vi "UpdateData_Wrapper.vi"(6 "50mA Spectra":cluster{"Wavelength":dbl[], "EL Spectrum":dbl[]}, 7 "20mA Spectra":cluster{"Wavelength":dbl[], "EL Spectrum":dbl[]}, 8 "error in (no error)":errorcluster, 10 "Data In":T1 {"50mA Data"."Reverse" format="%#_3g"; "50mA Data"."Current,mA" format="%_6g"; "50mA Data"."Knee Current" format="%#_3g"; "50mA Data"."WL" format="%_6g"; "50mA Data"."Voltage" format="%_6g"; "50mA Data"."Power" format="%_5g"; "20mA Data"."Reverse" format="%#_3g"; "20mA Data"."Current,mA" format="%_6g"; "20mA Data"."Knee Current" format="%#_3g"; "20mA Data"."WL" format="%_6g"; "20mA Data"."Voltage" format="%_6g"; "20mA Data"."Power" format="%_5g"}, 11 "EpiWrapper in":refnum<class "EpiWrapper.lvclass">) -> (0 "error out":errorcluster, 1 "PowerMin":dbl, 2 "KneeFail?":bool, 3 "EpiWrapper out":refnum<class "EpiWrapper.lvclass">)   [LabVIEW 2012, in "EpiWrapper.lvclass"]
uses:
  EpiWrapper.lvclass
  Controls/TestData.ctl
  Controls/Measurement.ctl
  EpiWrapper.lvclass/EpiWrapper.ctl
  LotData.lvclass
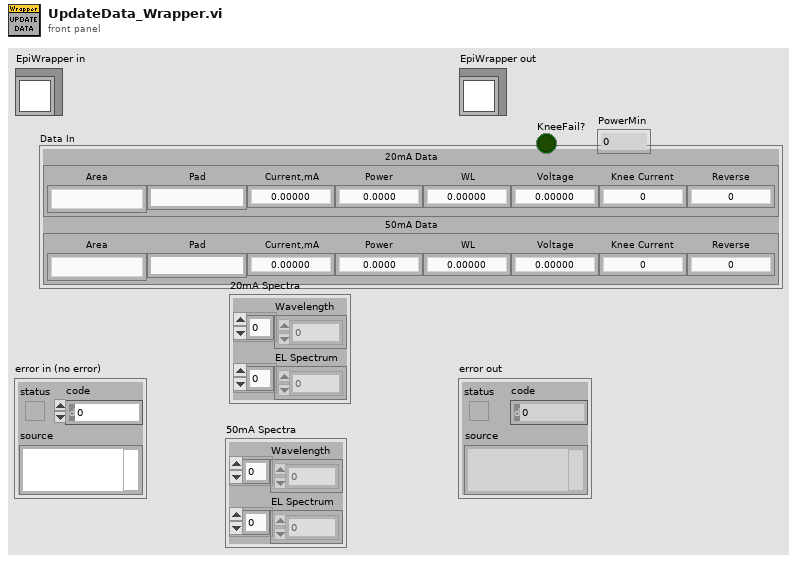
[diagram p1: front panel]
types:
  T1 = typedef "TestData.ctl" = cluster{"20mA Data":T2, "50mA Data ":T2}
  T2 = typedef "Measurement.ctl" = cluster{"Area":string, "Pad":string, "Current,mA":dbl, "Power":dbl, "WL":dbl, "Voltage":dbl, "Knee Current":dbl, "Reverse":dbl}
  T3 = typedef "Config.ctl" = cluster{"IntTime":i32, "Samples":i32, "PowerMin":dbl, "KneeMin":dbl, "KneeMax":dbl, "Background Wl":dbl, "Settle Delay,ms":u32, "StationId":sgl}
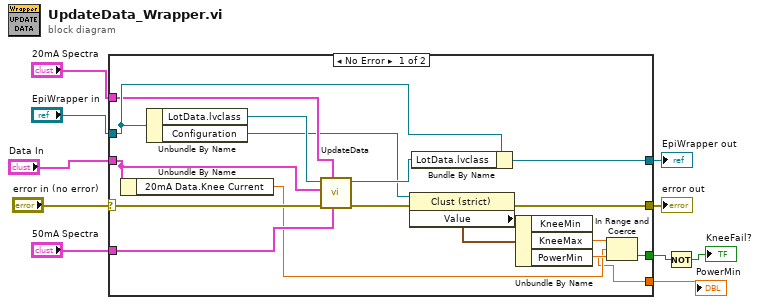
[diagram p0: block diagram]
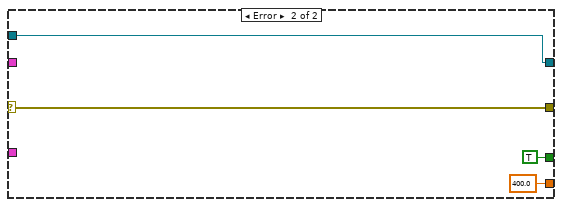
[diagram p2: hidden frame]
diagram:
  n1 = case shown="No Error" "error in (no error)" {
    selector: "error in (no error)" -> [w24 w31]
    tunnel: [w12 w31] -> w9
    tunnel: [w22 w30] -> w7
    tunnel: "EpiWrapper in" -> [w26 w30]
    tunnel: "Data In" -> [w18 _]
    tunnel: "20mA Spectra" -> [w23 _]
    tunnel: "50mA Spectra" -> [w21 _]
    tunnel: [w14 TRUE] -> w3
    tunnel: [w11 400.0 ("PowerMin")] -> w1
    frame No Error {
      n2 = Unbundle By Name(w18) -> ("20mA Data.Knee Current"=w15:dbl)
      n3 = Unbundle By Name(w26) -> ("LotData.lvclass"=w27:refnum<class "LotData.lvclass">, "Configuration"=w20:refnum<vi>)
      n4 = call-dynamic "UpdateData.vi"("50mA Spectra"=w21, "20mA Spectra"=w23, "error in (no error)"=w24, "Data In"=w18, "LotData in"=w27) -> ("error out"=w13:errorcluster, "LotData out"=w25:refnum<class "LotData.lvclass">)  [unwired: 4 in, 1 out]
      n5 = property class="Clust (strict)"(reference=w20, error in=w13) -> (error out=w12:errorcluster, "Value"=w19:T3)  [unwired: 1 out]
      n6 = Bundle By Name(cluster=w26, "LotData.lvclass"=w25) -> (w22:refnum<class "EpiWrapper.lvclass">)
      n7 = Unbundle By Name(w19) -> ("KneeMin"=w16:dbl, "KneeMax"=w17:dbl, "PowerMin"=w11:dbl)
      n8 = In Range and Coerce(upper limit=w17, x=w15, lower limit=w16) -> (In Range?=w14:bool)  [unwired: 1 out]
    }
    frame Error {
    }
  }
  "error out" <- w9
  "EpiWrapper out" <- w7
  "PowerMin" <- w1
  n9 = Not(x=w3) -> (.not. x?=→"KneeFail?":bool)
